vi "d6.6 (hw6).vi"() -> ()   [LabVIEW 2017]
panel:
  out "Min":dbl
  out "Max":dbl
  out "Array Size":dbl
  out "SubArray":dbl[](array[numeric])
  out "Array Size":dbl
  out "Array Size":dbl
  out "Array Sorted":dbl[](array[numeric])
  out "Array Unsorted":dbl[](array[numeric])
  in  "n - input":dbl
  # "Overview: This VI will be given an input of n and make two array's of that size made up of random numbers. Currently the arrays are set to size 5 but you can parse through the index using the index scroller to the left of each array for any array larger than 5. The second array is sorted, smallest to largest in ascending order. The third is a subarray only consisting of elements 2 and 3 (Sorted array).\n\nPatrik Sokolowski\n\nHW 7 (D6.6) modified"
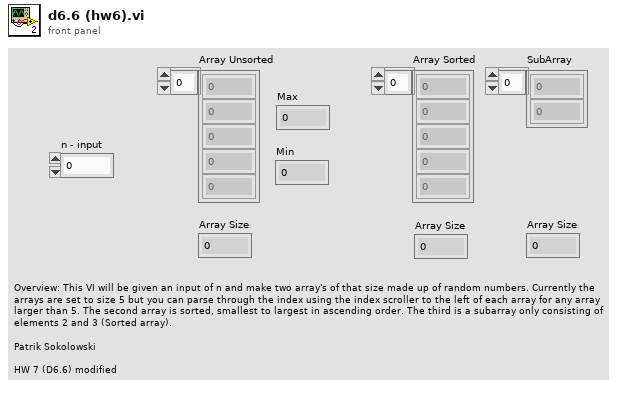
[diagram p1: front panel]
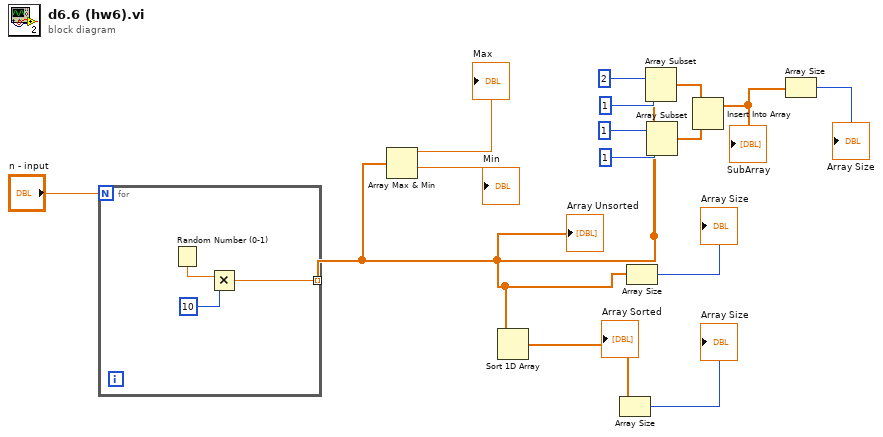
[diagram p0: block diagram]
diagram:
  n1 = for {
    N: "n - input" -> [_]
    tunnel: [w16] -> w1 mode=indexing
    n2 = Random Number (0-1)() -> (number: 0 to 1=w18:dbl)
    n3 = Multiply(x=w18, y=10) -> (x*y=w16:dbl)
  }
  "Array Unsorted" <- w1
  n4 = Array Max & Min(array=w1) -> (max value=→"Max":dbl, min value=→"Min":dbl)  [unwired: 2 out]
  n5 = Sort 1D Array(array=w1) -> (sorted array=w14:dbl[])
  "Array Sorted" <- w14
  n6 = Array Size(array=w14) -> (size(s)=→"Array Size":i32)
  n7 = Array Size(array=w1) -> (size(s)=→"Array Size":i32)
  n8 = Array Subset(array=w1, index=2, length=1) -> (w7:dbl[])
  n9 = Array Subset(array=w1, index=1, length=1) -> (w6:dbl[])
  n10 = Insert Into Array(array=w6, new element=w7) -> (w5:dbl[])  [unwired: 1 in]
  "SubArray" <- w5
  n11 = Array Size(array=w5) -> (size(s)=→"Array Size":i32)
